vi "Periodic Tasks.vi"(8 "error in":errorcluster) -> ()   [LabVIEW 2018]
doc: "This VI runs in parallel to other tasks. It can contain as many user-defined periodic loops as you need. These can carry out PID or other sorts of timed response."
uses:
  State Machines/Intake.ctl
  State Machines/Climber.ctl
  <vilib>/Rock Robotics/WPI/Solenoid/WPI_SolenoidValue.ctl
  <vilib>/Rock Robotics/WPI/ThirdParty/Phoenix-LabVIEW/Motor Controller/Controls/CTRE_Phoenix_MotorControl_ControlMode.ctl
  <vilib>/Rock Robotics/WPI/ThirdParty/Sensors/navX/_TypeDefs/FRIC_navX_DeviceNumbersTypeDef.ctl
  <vilib>/Rock Robotics/WPI/DriverStation/WPI_DriverStationRobotMode2.ctl
  Robot Global Data.vi
  Support Code/Valkyrie1Buttons.vi
  <vilib>/Rock Robotics/WPI/Utilities/WPI_GetSetVariantRefNum.vi
  <vilib>/Rock Robotics/WPI/Solenoid/WPI_SolenoidSetEnum.vi
  <vilib>/Rock Robotics/Network Tables/NT Write Number.vi
  <vilib>/Rock Robotics/Network Tables/NT Write Boolean.vi
panel:
  in  "ScoreHatchHeight":dbl=1.0
  in  "HP_Height":dbl=1.5
  in  "HatchGetSpeed":dbl=-1.0
  in  "SetpointElevatorCargo":dbl=5.5
  in  "ElevatorCargoDelay":dbl
  in  "Delay Cargo IR":dbl=5.0
  in  "Time to wait":dbl
  in  "Back Timer":dbl=15.0 format="%#_13g"
  in  "Retract back Speed 2":dbl=-0.4 format="%#_13g"
  in  "Retract Speed 2":dbl=-0.3
  in  "Retract Distance 2":dbl=700.0 format="%#_13g"
  in  "Back Speed 2":dbl=0.8
  in  "Front Speed 2":dbl=1.0
  in  "Front Limit 2":dbl=700.0 format="%#_13g"
  in  "Break speed 2":dbl=0.2 format="%#_13g"
  out "Climber State 2":T1=enum."Wait for Start"
  in  "Climb Height":dbl=2.0
  in  "Score Hatch Angle 2":dbl=2.0
  out "Climber State":T1=enum."Wait for Start"
  in  "Retract back Speed":dbl=-0.4 format="%#_13g"
  in  "Retract Distance":dbl=1750.0 format="%#_13g"
  in  "Retract Speed":dbl=-0.3
  in  "Break speed":dbl=0.2 format="%#_13g"
  in  "Front Limit":dbl=1750.0 format="%#_13g"
  in  "Front Speed":dbl=1.0
  in  "Back Speed":dbl=0.75
  out "Encoder Climber":i32
  in  "Score Angle 2nd":dbl=3.0
  in  "Slow Mode":dbl=0.4
  in  "Cargo Deploy angle 2nd Floor":dbl=5.0
  in  "Cargo 2nd Floor Rocket":dbl=9.5
  in  "Cargo ship height":dbl=9.0
  in  "Cargo 1st Floor Rocket":dbl=5.0 format="%#_13g"
  out "elavador  pos":dbl
  in  "Height  Hatch 2nd":dbl=9.0
  out "Intake pos":dbl=23.023681640625
  in  "Turn on point multiplier":dbl=0.6 format="%#_13g"
  in  "Sensitivty":dbl=1.1 format="%#_13g"
  in  "Height Cargo Station":dbl=2.0
  in  "Height Cargo HP":dbl=9.0
  in  "Floor Angle Cargo":dbl=22.0
  in  "Gains":T2={"proportional gain (Kc)"=0.5, "integral time (Ti, min)"=0.1, "derivative time (Td, min)"=0.0} {"derivative time (Td, min)" format="%.3f"; "integral time (Ti, min)" format="%.3f"; "proportional gain (Kc)" format="%.3f"}
  in  "Range":cluster{"output high":dbl, "output low":dbl}={"output high"=1.0, "output low"=-0.4} {"output low" format="%.2f"; "output high" format="%.2f"}
  in  "Disable Range":dbl
  in  "Integral Range":dbl=1.0
  in  "CargoTime":dbl=10.0
  in  "Default height":dbl=3.0 format="%#_13g"
  in  "Cargo Deploy Angle":dbl=15.0
  in  "Tempo de coleta":dbl=7.0 format="%#_13g"
  out "Estado Intake":T3
  in  "Score Hatch Angle":dbl=2.0 format="%#_13g"
  in  "Floor Angle":dbl=23.0
  in  "Hatch intake Speed Floor":dbl=-1.0
  in  "Holding Angle":dbl=4.0
  in  "HP Angle":dbl=1.0 format="%#_13g"
  in  "Intake Arm PID Constants":T4={"P Gain"=0.15, "I Gain"=1e-05, "D Gain"=5.0, "F Gain"=0.0, "I Zone"=10.0, "Min Output"=-0.2999999999999998, "Max Output"=0.3} {"Max Output" min=-1.0 max=1.0 step=0.01; "Min Output" min=-1.0 max=1.0 step=0.01; "I Zone" step=0.01; "F Gain" step=0.01; "D Gain" step=0.01; "I Gain" step=0.01; "P Gain" min=0.0 step=0.01}
  # "Angles"
  # "Intake Control"
  # "Elevator Control"
  # "Climber"
  # "Drivetrain"
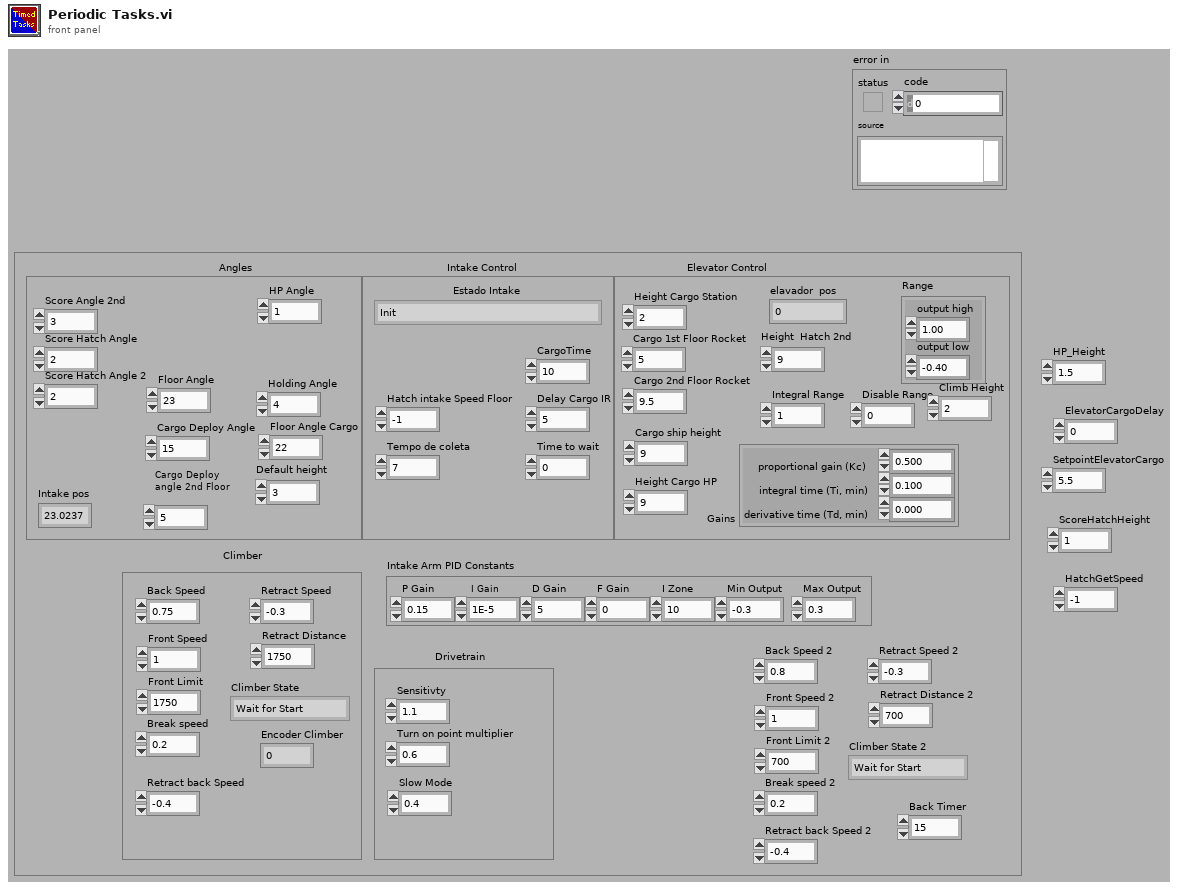
[diagram p1: front panel]
types:
  T1 = typedef "Climber.ctl" = enum16{"Engaging Climb", "Wait for Start", "ELEVATE!", "Hold position", "Forward", "Retract varetas", "Charge", "Sobe so um poquinho", "cabou"}
  T2 = cluster{"proportional gain (Kc)":dbl, "integral time (Ti, min)":dbl, "derivative time (Td, min)":dbl}
  T3 = typedef "Intake.ctl" = enum16{"Init", "Preparar Coletar HP", "Coletar Cargo", "Segurando Cargo", "Preparar Score Cargo", "Score Cargo", "Coletar HP", "Coletar Hatch Chão", "Segurando Hatch", "Preparar Score Hatch", "Score Hatch", "Wait"}
  T4 = cluster{"P Gain":dbl, "I Gain":dbl, "D Gain":dbl, "F Gain":dbl, "I Zone":dbl, "Min Output":dbl, "Max Output":dbl}
  T5 = typedef "WPI_MotorControlDeviceRef.ctl" = cluster{"DeviceStatus":errorcluster, "Type":T6, "PWM":cluster{"PWM Channel":T7, "DeadBand":T8}, "CAN":cluster{"Device Number":u8, "SetOutput VI Ref":variant, "GetOutput VI Ref":variant, "Enable VI Ref":variant, "Disable VI Ref":variant, "Data":variant}, "Invert":bool, "DIO PWM":cluster{"PWM \"Enable\" Channel":T7, "DIOChannel":T9, "PWM Rate":dbl}}
  T6 = typedef "WPI_MotorControlType.ctl" = enum16{"PWM", "CAN", "DIO PWM"}
  T7 = typedef "FPGA_DIOPWMChannel.ctl" = enum8{"PWM 0", "PWM 1", "PWM 2", "PWM 3", "PWM 4", "PWM 5", "PWM 6", "PWM 7", "PWM 8", "PWM 9", "PWM MXP 0", "PWM MXP 1", "PWM MXP 2", "PWM MXP 3", "PWM MXP 4", "PWM MXP 5", "PWM MXP 6", "PWM MXP 7", "PWM MXP 8", "PWM MXP 9", "Invalid"}
  T8 = typedef "WPI_PWMDeadband.ctl" = cluster{"Name":string, "maxPositivePwm":i32, "minPositivePwm":i32, "centerPwm":i32, "maxNegativePwm":i32, "minNegativePwm":i32, "angularRange":u16}
  T9 = typedef "FPGA_DIOChannel.ctl" = enum8{"DIO 0", "DIO 1", "DIO 2", "DIO 3", "DIO 4", "DIO 5", "DIO 6", "DIO 7", "DIO 8", "DIO 9", "DIO MXP 0", "DIO MXP 1", "DIO MXP 2", "DIO MXP 3", "DIO MXP 4", "DIO MXP 5", "DIO MXP 6", "DIO MXP 7", "DIO MXP 8", "DIO MXP 9", "DIO MXP 10", "DIO MXP 11", "DIO MXP 12", "DIO MXP 13", "DIO MXP 14", "DIO MXP 15", "SPI Port CS1", "SPI Port CS2", "SPI Port CS3", "SPI Port MISO", "SPI Port MOSI", "Invalid"}
  T10 = typedef "Button Cluster.ctl" = cluster{"Buttons[0]":bool, "Buttons[1]":bool, "Buttons[2]":bool, "Buttons[3]":bool, "Buttons[4]":bool, "Buttons[5]":bool, "Buttons[6]":bool, "Buttons[7]":bool, "Buttons[8]":bool, "Buttons[9]":bool}
  T11 = typedef "WPI_SwitchDevRef.ctl" = cluster{"DevStatus":errorcluster, "DIO Channel":T9, "CntIndex":T12, "Normally Closed":bool}
  T12 = typedef "FPGA_CounterCtrSystemIndex.ctl" = enum8{"Ctr 0", "Ctr 1", "Ctr 2", "Ctr 3", "Ctr 4", "Ctr 5", "Ctr 6", "Ctr 7", "Invalid"}
  T13 = typedef "WPI_SolenoidDevRef.ctl" = cluster{"DevStatus":errorcluster, "Pneumatics Control Module":u8, "Forward Solenoid Channel":T14, "Reverse Solenoid Channel":T14}
  T14 = typedef "WPI_SolenoidChannel.ctl" = enum8{"Solenoid 0", "Solenoid 1", "Solenoid 2", "Solenoid 3", "Solenoid 4", "Solenoid 5", "Solenoid 6", "Solenoid 7", "Invalid"}
  T15 = typedef "WPI_EncoderDevRef.ctl" = cluster{"DevStatus":errorcluster, "EncoderIndex":T16, "CounterIndex":T12, "DistancePerCount":dbl, "Decoding Type":T17}
  T16 = typedef "FPGA_EncoderIdx.ctl" = enum8{"Enc 0", "Enc 1", "Enc 2", "Enc 3", "Enc 4", "Enc 5", "Enc 6", "Enc 7", "Invalid"}
  T17 = typedef "WPI_EncoderType.ctl" = enum16{"1x", "2x", "4x"}
  T18 = typedef "WPI_SolenoidValue.ctl" = enum16{"Off", "On", "Forward", "Reverse"}
  T19 = typedef "CTRE_Phoenix_MotorControl_ControlMode.ctl" = u16
  T20 = typedef "WPI_CounterDevRef.ctl" = cluster{"DevStatus":errorcluster, "CntIndex":T12}
  T21 = typedef "FRIC_navX_DeviceNumbersTypeDef.ctl" = enum16{"Dev0", "Dev1", "Dev2", "Dev3"}
  T22 = cluster{"Yaw":dbl, "Roll":dbl, "Pitch":dbl, "Heading":dbl, "Fused Heading":dbl}
  T23 = typedef "WPI_RobotDriveDevRef.ctl" = cluster{"DevStatus":errorcluster, "Motors[]":T5[], "Square Inputs":bool, "Max Output":dbl}
  T24 = typedef "Axes Cluster.ctl" = cluster{"Axes[0]":dbl, "Axes[1]":dbl, "Axes[2]":dbl, "Axes[3]":dbl, "Axes[4]":dbl, "Axes[5]":dbl, "Axes[6]":dbl, "Axes[7]":dbl, "Axes[8]":dbl}
  T25 = typedef "WPI_DriverStationRobotMode2.ctl" = enum16{"Autonomous Disabled", "Autonomous Enabled", "Teleop Disabled", "Teleop Enabled", "Disconnected", "Finish", "Test Disabled", "Test Enabled", "Emergency Stopped"}
  T26 = typedef "WPI_CompressorDevRef.ctl" = cluster{"DevStatus":errorcluster, "Pneumatics Control Module":u8}
  T27 = typedef "WPI_JoystickDevRef.ctl" = cluster{"Device":T28}
  T28 = typedef "WPI_JoystickDeviceEnum.ctl" = enum16{"USB 0", "USB 1", "USB 2", "USB 3", "USB 4", "USB 5"}
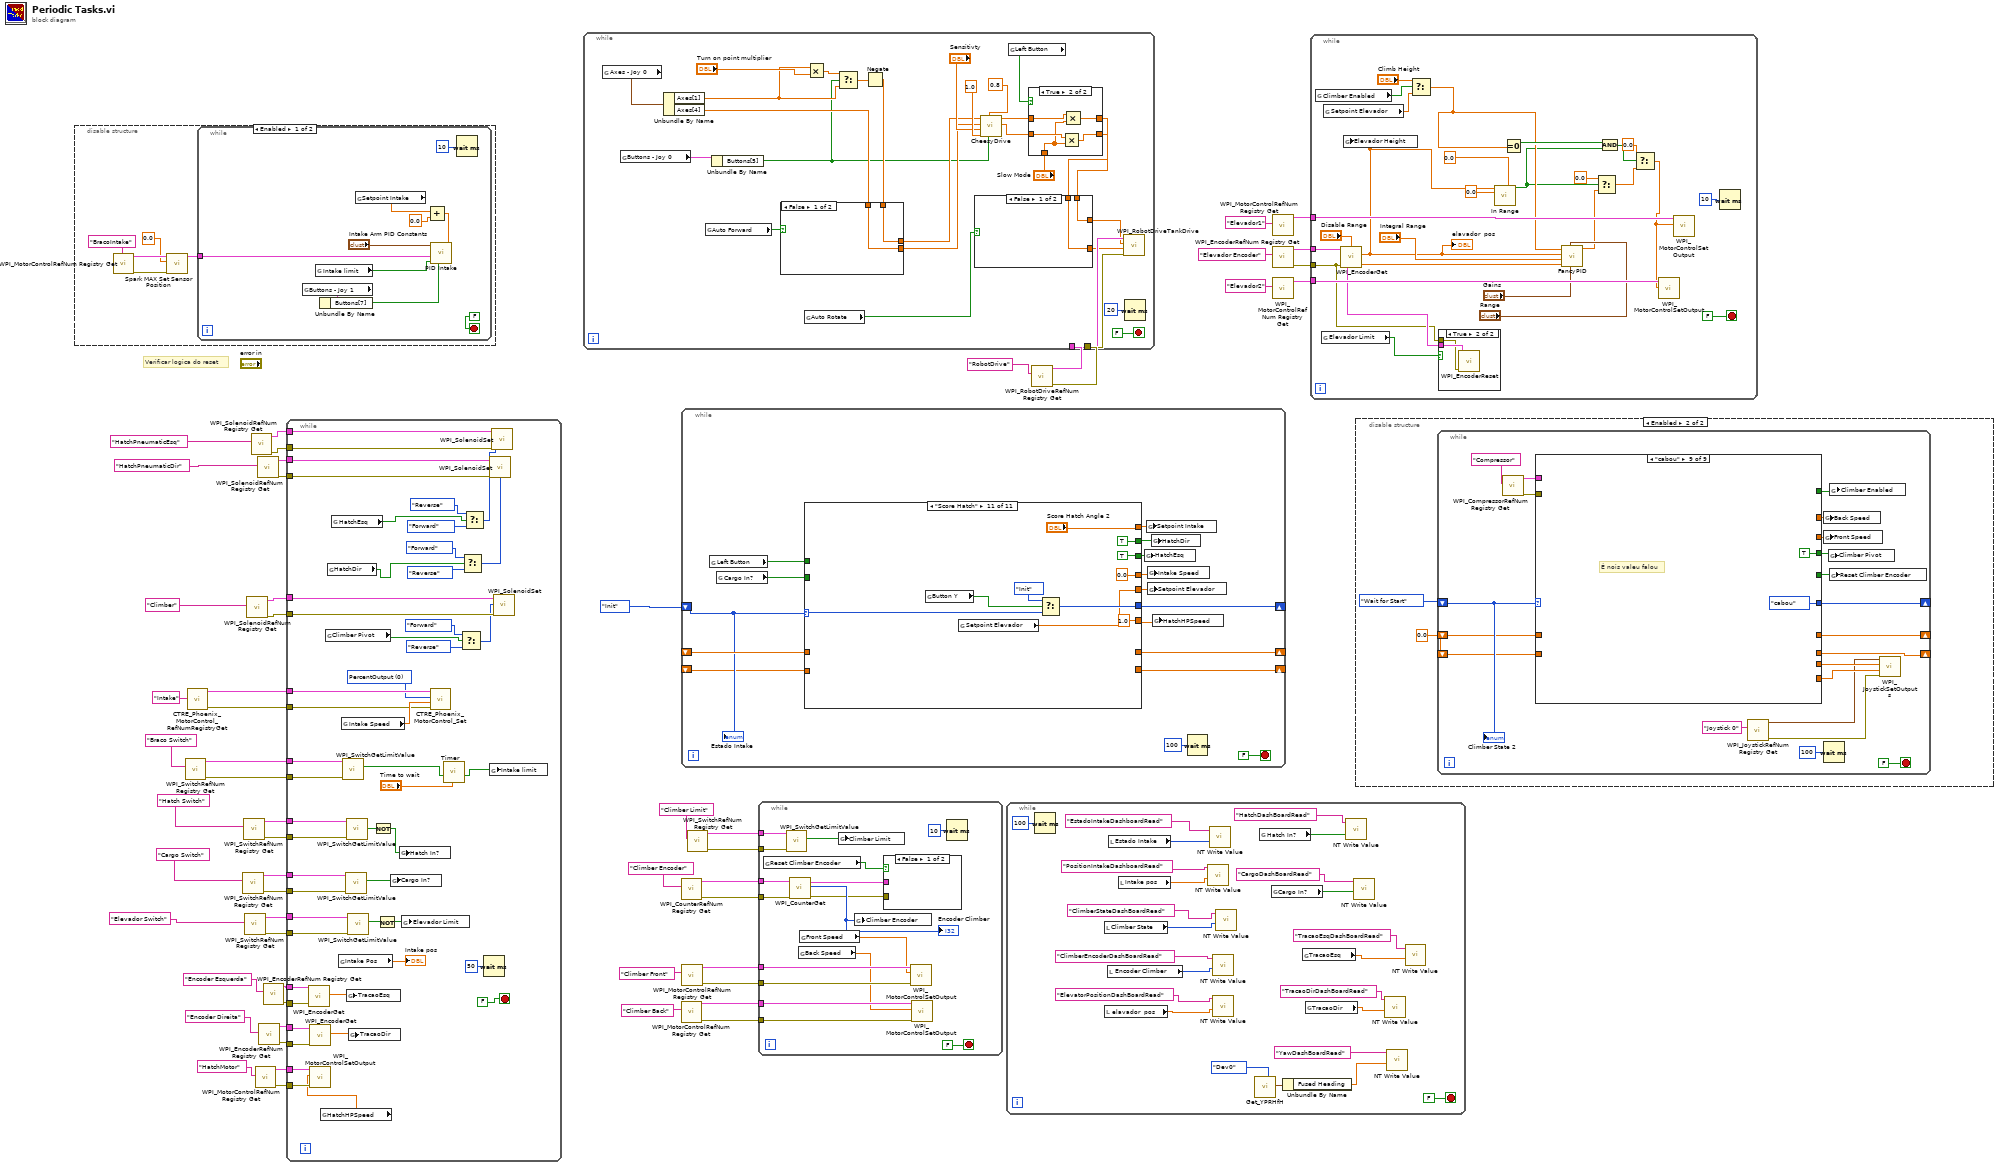
[diagram p0: block diagram]
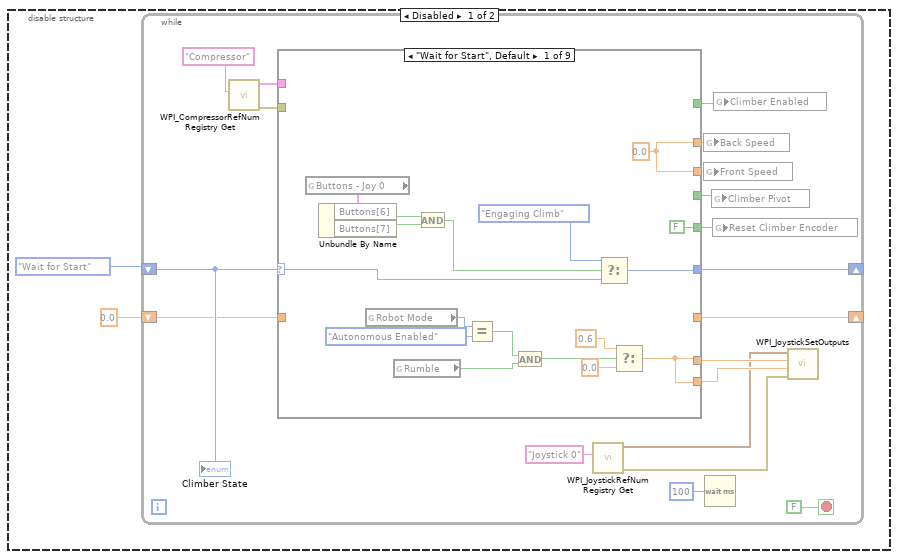
[diagram p2: hidden frame]
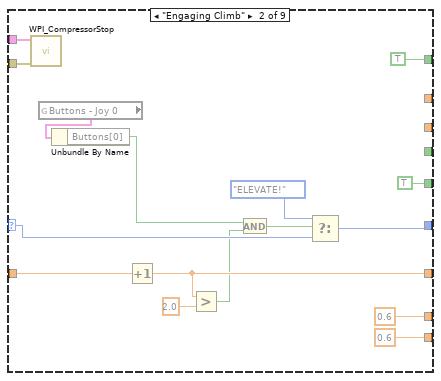
[diagram p3: hidden frame]
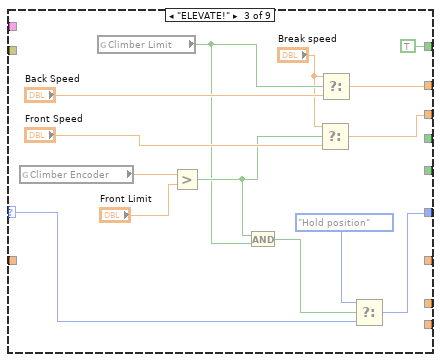
[diagram p4: hidden frame]
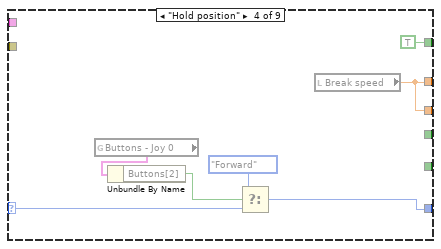
[diagram p5: hidden frame]
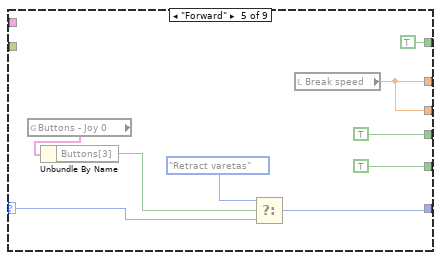
[diagram p6: hidden frame]
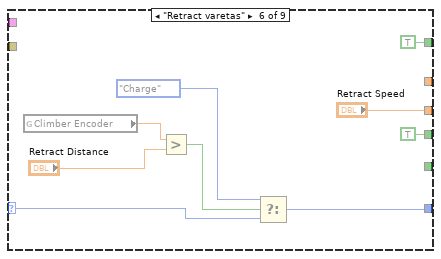
[diagram p7: hidden frame]
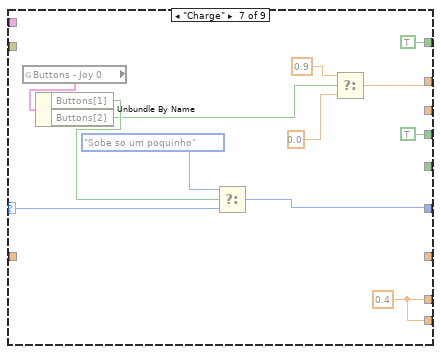
[diagram p8: hidden frame]
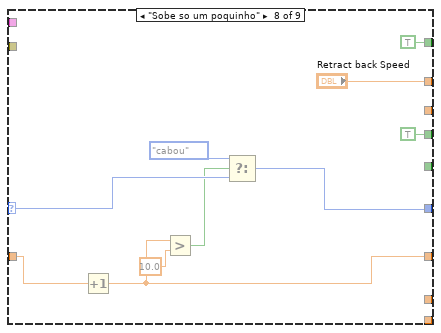
[diagram p9: hidden frame]
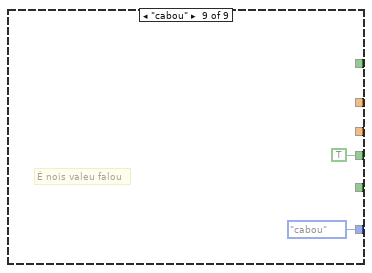
[diagram p10: hidden frame]
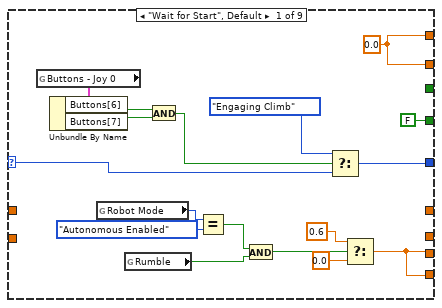
[diagram p11: hidden frame]
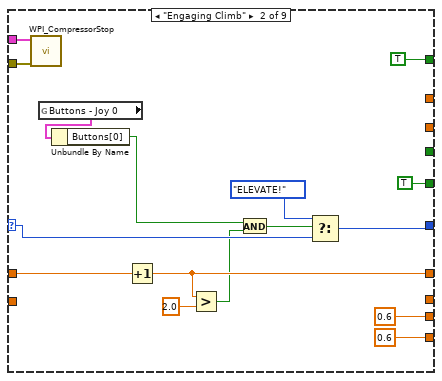
[diagram p12: hidden frame]
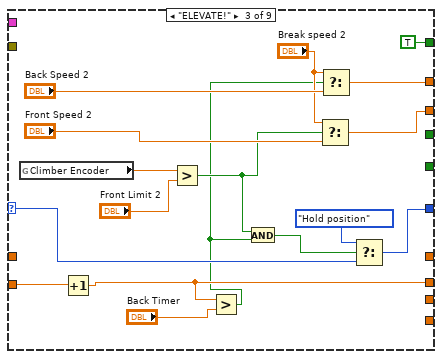
[diagram p13: hidden frame]
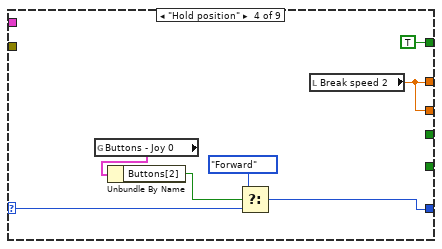
[diagram p14: hidden frame]
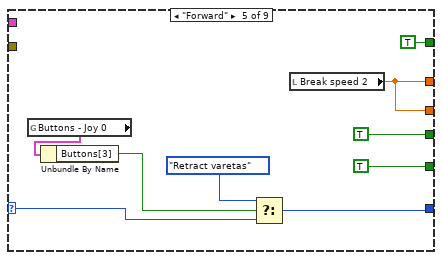
[diagram p15: hidden frame]
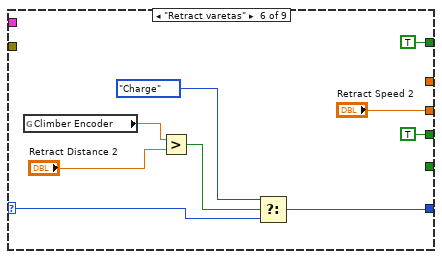
[diagram p16: hidden frame]
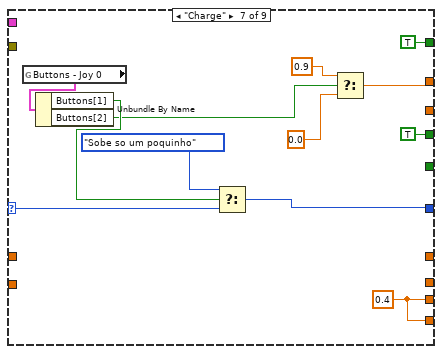
[diagram p17: hidden frame]
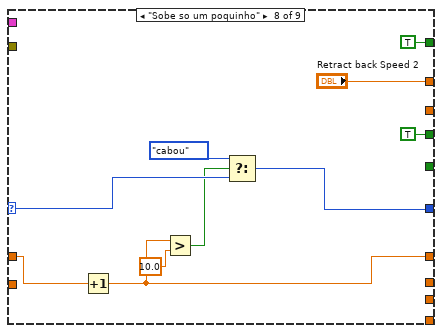
[diagram p18: hidden frame]
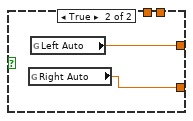
[diagram p20: hidden frame]
diagram:
  # "Verificar logica do reset"
  n1 = disable-structure shown="Enabled" {
    frame Enabled {
      n2 = call <vilib>:"WPI_MotorControlRefNum Registry Get.vi"("refnum name"="BracoIntake") -> ("error out"=w58:errorcluster, "MotorControlDevRef"=w59:T5)  [unwired: 9 in]
      n3 = call <vilib>:"Spark MAX Set Sensor Position.vi"("error in"=w58, "Position"=0.0, "MotorControlDeviceRef"=w59) -> ("MotorControlDeviceRef"=w60:T5)  [unwired: 7 in, 1 out]
      n4 = while {
        tunnel: w60 -> [w69]
        stop <- FALSE stop-if-true
        n5 = global read "Robot Global Data.vi" "Buttons - Joy 1"() -> (w67:T10)
        n6 = global read "Robot Global Data.vi" "Intake limit"() -> (w65:bool)
        n7 = Unbundle By Name(w67) -> ("Buttons[7]"=w66:bool)
        n8 = global read "Robot Global Data.vi" "Setpoint Intake"() -> (w64:dbl)
        n9 = Add(x=w64, y=0.0) -> (x+y=w63:dbl)
        n10 = call "PID Intake.vi"("Encoder Overide"=w66, "Limit"=w65, "Setpoint Intake"=w63, "MotorControlDevRef"=w69, "PID Constants"="Intake Arm PID Constants") -> ()  [unwired: 7 in]
        n11 = Wait (ms)(milliseconds to wait=u32 10) -> ()  [unwired: 1 out]
      }
    }
    frame Disabled {
    }
  }
  n12 = call <vilib>:"WPI_SwitchRefNum Registry Get.vi"("refnum name"="Braco Switch") -> ("error out"=w52:errorcluster, "SwitchDevRef"=w53:T11)  [unwired: 9 in]
  n13 = call <vilib>:"CTRE_Phoenix_MotorControl_RefNumRegistryGet.vi"("refnum name"="Intake") -> ("error out"=w48:errorcluster, "PhoenixMotorControlDevRef"=w49:T5)  [unwired: 9 in]
  n14 = call <vilib>:"WPI_SwitchRefNum Registry Get.vi"("refnum name"="Cargo Switch") -> ("error out"=w39:errorcluster, "SwitchDevRef"=w40:T11)  [unwired: 9 in]
  n15 = call <vilib>:"WPI_SwitchRefNum Registry Get.vi"("refnum name"="Hatch Switch") -> ("error out"=w47:errorcluster, "SwitchDevRef"=w46:T11)  [unwired: 9 in]
  n16 = call <vilib>:"WPI_SwitchRefNum Registry Get.vi"("refnum name"="Elevador Switch") -> ("error out"=w27:errorcluster, "SwitchDevRef"=w26:T11)  [unwired: 9 in]
  n17 = call <vilib>:"WPI_SolenoidRefNum Registry Get.vi"("refnum name"="Climber") -> ("error out"=w43:errorcluster, "SolenoidDevRef"=w42:T13)  [unwired: 9 in]
  n18 = call <vilib>:"WPI_SolenoidRefNum Registry Get.vi"("refnum name"="HatchPneumaticEsq") -> ("error out"=w37:errorcluster, "SolenoidDevRef"=w36:T13)  [unwired: 9 in]
  n19 = call <vilib>:"WPI_MotorControlRefNum Registry Get.vi"("refnum name"="HatchMotor") -> ("error out"=w2:errorcluster, "MotorControlDevRef"=w3:T5)  [unwired: 9 in]
  n20 = call <vilib>:"WPI_SolenoidRefNum Registry Get.vi"("refnum name"="HatchPneumaticDir") -> ("error out"=w54:errorcluster, "SolenoidDevRef"=w55:T13)  [unwired: 9 in]
  n21 = call <vilib>:"WPI_EncoderRefNum Registry Get.vi"("refnum name"="Encoder Direita") -> ("error out"=w4:errorcluster, "EncoderDevRef"=w5:T15)  [unwired: 9 in]
  n22 = call <vilib>:"WPI_EncoderRefNum Registry Get.vi"("refnum name"="Encoder Esquerda") -> ("error out"=w7:errorcluster, "EncoderDevRef"=w8:T15)  [unwired: 9 in]
  n23 = while {
    tunnel: w36 -> [w121]
    tunnel: w37 -> [w120]
    tunnel: w55 -> [w119]
    tunnel: w54 -> [w118]
    tunnel: w42 -> [w117]
    tunnel: w43 -> [w116]
    tunnel: w49 -> [w104]
    tunnel: w53 -> [w101]
    tunnel: w52 -> [w100]
    tunnel: w48 -> [w99]
    tunnel: w46 -> [w97]
    tunnel: w47 -> [w98]
    tunnel: w40 -> [w93]
    tunnel: w39 -> [w92]
    tunnel: w26 -> [w87]
    tunnel: w27 -> [w88]
    tunnel: w7 -> [w84]
    tunnel: w5 -> [w82]
    tunnel: w4 -> [w81]
    tunnel: w8 -> [w79]
    tunnel: w3 -> [w74]
    tunnel: w2 -> [w73]
    stop <- FALSE stop-if-true
    w103 = T19 0 items=["PercentOutput"=0, "Position"=1, "Velocity"=2, "Current"=3, "Follower"=5, "MotionProfile"=6, "MotionMagic"=7, "MotionProfileArc"=10, "Disabled"=15] ("Control Mode")
    n24 = call <vilib>:"WPI_EncoderGet.vi"("error in (no error)"=w84, "EncoderDevRef"=w79) -> ("Distance"=w83:dbl)  [unwired: 4 in, 5 out]
    n25 = call <vilib>:"WPI_EncoderGet.vi"("error in (no error)"=w81, "EncoderDevRef"=w82) -> ("Distance"=w80:dbl)  [unwired: 4 in, 5 out]
    n26 = global read "Robot Global Data.vi" "HatchHPSpeed"() -> (w72:dbl)
    n27 = call <vilib>:"WPI_MotorControlSetOutput.vi"("error in (no error)"=w73, "Output"=w72, "MotorControlDevRef"=w74) -> ()  [unwired: 6 in, 3 out]
    n28 = global read "Robot Global Data.vi" "Climber Pivot"() -> (w105:bool)
    n29 = global read "Robot Global Data.vi" "HatchDir"() -> (w95:bool)
    n30 = global read "Robot Global Data.vi" "HatchEsq"() -> (w94:bool)
    n31 = global read "Robot Global Data.vi" "Intake Pos"() -> (→"Intake pos":dbl)
    n32 = global read "Robot Global Data.vi" "Intake Speed"() -> (w102:dbl)
    n33 = call <vilib>:"WPI_SwitchGetLimitValue.vi"("error in (no error)"=w100, "SwitchDevRef"=w101) -> ("Switch Pressed"=w77:bool)  [unwired: 7 in, 2 out]
    n34 = call <vilib>:"WPI_SwitchGetLimitValue.vi"("error in (no error)"=w92, "SwitchDevRef"=w93) -> ("Switch Pressed"=w85:bool)  [unwired: 7 in, 2 out]
    n35 = call <vilib>:"WPI_SwitchGetLimitValue.vi"("error in (no error)"=w98, "SwitchDevRef"=w97) -> ("Switch Pressed"=w96:bool)  [unwired: 7 in, 2 out]
    n36 = global write "Robot Global Data.vi" "TracaoEsq"(w83) -> ()
    n37 = call <vilib>:"WPI_SwitchGetLimitValue.vi"("error in (no error)"=w88, "SwitchDevRef"=w87) -> ("Switch Pressed"=w89:bool)  [unwired: 7 in, 2 out]
    n38 = global write "Robot Global Data.vi" "TracaoDir"(w80) -> ()
    n39 = Not(x=w96) -> (.not. x?=w91:bool)
    n40 = Not(x=w89) -> (.not. x?=w86:bool)
    n41 = global write "Robot Global Data.vi" "Cargo In?"(w85) -> ()
    n42 = global write "Robot Global Data.vi" "Hatch In?"(w91) -> ()
    n43 = global write "Robot Global Data.vi" "Elevador Limit"(w86) -> ()
    n44 = call <vilib>:"CTRE_Phoenix_MotorControl_Set.vi"("error in (no error)"=w99, "Output"=w102, "Control Mode"=w103, "PhoenixMotorControlDevRef"=w104) -> ()  [unwired: 6 in, 2 out]
    n45 = call "Timer.vi"("Timer to wait"="Time to wait", "Switch Pressed"=w77) -> ("Out"=w76:bool)  [unwired: 9 in]
    n46 = Select(t=WPI_SolenoidValue."Forward" ("Value"), s=w105, f=WPI_SolenoidValue."Reverse") -> (s? t:f=w111:T18)
    n47 = Select(t=WPI_SolenoidValue."Forward" ("Value"), s=w95, f=WPI_SolenoidValue."Reverse") -> (s? t:f=w108:T18)
    n48 = Select(t=WPI_SolenoidValue."Reverse" ("Value"), s=w94, f=WPI_SolenoidValue."Forward") -> (s? t:f=w75:T18)
    n49 = Wait (ms)(milliseconds to wait=u32 50) -> ()  [unwired: 1 out]
    n50 = call-poly <vilib>:"WPI_SolenoidSet.vi"("error in (no error)"=w118, "Value"=w108, "SolenoidDevRef"=w119) -> ()  [unwired: 7 in, 2 out]
    n51 = global write "Robot Global Data.vi" "Intake limit"(w76) -> ()
    n52 = call-poly <vilib>:"WPI_SolenoidSet.vi"("error in (no error)"=w120, "Value"=w75, "SolenoidDevRef"=w121) -> ()  [unwired: 7 in, 2 out]
    n53 = call-poly <vilib>:"WPI_SolenoidSet.vi"("error in (no error)"=w116, "Value"=w111, "SolenoidDevRef"=w117) -> ()  [unwired: 7 in, 2 out]
  }
  n54 = call <vilib>:"WPI_CounterRefNum Registry Get.vi"("refnum name"="Climber Encoder") -> ("error out"=w19:errorcluster, "CounterDevRef"=w20:T20)  [unwired: 9 in]
  n55 = call <vilib>:"WPI_MotorControlRefNum Registry Get.vi"("refnum name"="Climber Back") -> ("error out"=w13:errorcluster, "MotorControlDevRef"=w15:T5)  [unwired: 9 in]
  n56 = while {
    shift-right: [w136] -> _
    shift-left: Intake."Init" -> [w132]
    shift-right: [w133] -> _
    shift-left: _ -> [w134]
    shift-right: [w131] -> _
    shift-left: _ -> [w130]
    stop <- FALSE stop-if-true
    n57 = global read "Valkyrie1Buttons.vi" "Left Button"() -> (w123:bool)
    n58 = global read "Robot Global Data.vi" "Cargo In?"() -> (w124:bool)
    n59 = case shown="\"Score Hatch\"" w132 {
      selector: w132 -> [w162 w178 w202 w219 w233 w256 w263 w272 w286 w310 w319]
      tunnel: [w142 "Floor Angle Cargo" w195 w207 w239 "HP Angle" _ "Floor Angle" "Holding Angle" w299 "Score Hatch Angle 2"] -> w129
      tunnel: [FALSE FALSE FALSE FALSE FALSE TRUE FALSE FALSE TRUE TRUE TRUE] -> w128
      tunnel: [FALSE FALSE FALSE FALSE FALSE TRUE FALSE FALSE TRUE TRUE TRUE] -> w127
      tunnel: [w151 w179 w192 w205 w235 w254 w266 w275 w290 w307 w318] -> w136
      tunnel: w134 -> [_ _ _ _ w230 w246 _ _ _ _ _]
      tunnel: [_ _ _ _ w228 w251 _ _ _ _ _] -> w133
      tunnel: [0.0 ("Hatch intake Speed Floor") 1.0 ("Hatch intake Speed Floor") w201 0.0 ("Hatch intake Speed Floor") -1.0 ("Hatch intake Speed Floor") 0.0 ("Hatch intake Speed Floor") _ "Hatch intake Speed Floor" 0.0 ("Hatch intake Speed Floor") 0.0 ("Hatch intake Speed Floor") 0.0 ("Hatch intake Speed Floor")] -> w126
      tunnel: w123 -> [w143 _ w188 _ _ _ _ w269 w283 _ _]
      tunnel: [_ _ _ _ _ 0.0 ("y") w259 _ _ _ _] -> w131
      tunnel: w130 -> [_ _ _ _ _ _ w260 _ _ _ _]
      tunnel: [0.0 ("ElevadorRocket") w187 0.0 ("ElevadorRocket") w212 w231 "HP_Height" 0.0 ("ElevadorRocket") 0.0 ("ElevadorRocket") 0.0 ("ElevadorRocket") w302 w313] -> w125
      tunnel: w124 -> [w148 w170 w200 _ _ _ _ _ _ _ _]
      tunnel: [_ _ _ _ _ "HatchGetSpeed" 0.1 ("HatchGetSpeed") 0.1 ("HatchSpeed") w281 -0.1 ("HatchGetSpeed") 1.0 ("HatchGetSpeed")] -> w122
      frame "Init", Default {
        n60 = global read "Valkyrie1Buttons.vi" "Button A"() -> (w152:bool)
        n61 = global read "Valkyrie1Buttons.vi" "Button X"() -> (w154:bool)
        n62 = global read "Valkyrie1Buttons.vi" "Button B"() -> (w153:bool)
        n63 = call "Timer.vi"("Timer to wait"="Delay Cargo IR", "Switch Pressed"=w143) -> ("Out"=w144:bool)  [unwired: 9 in]
        n64 = global read "Robot Global Data.vi" "Elevador Height"() -> (w139:dbl)
        n65 = Select(t=Intake."Preparar Coletar HP", s=w152, f=w162) -> (s? t:f=w161:T3)
        n66 = Select(t=Intake."Coletar Hatch Chão", s=w154, f=w161) -> (s? t:f=w156:T3)
        n67 = Less?(x=w139, y=6.0) -> (x < y?=w141:bool)
        n68 = Select(t=Intake."Coletar Cargo", s=w153, f=w156) -> (s? t:f=w150:T3)
        n69 = Select(t="Default height", s=w141, f=4.0) -> (s? t:f=w142:dbl)
        n70 = Select(t=Intake."Segurando Hatch", s=w144, f=w150) -> (s? t:f=w149:T3)
        n71 = Select(t=Intake."Segurando Cargo", s=w148, f=w149) -> (s? t:f=w151:T3)
      }
      frame "Coletar Cargo" {
        n72 = global read "Robot Global Data.vi" "Intake Pos"() -> (w168:dbl)
        n73 = global read "Valkyrie1Buttons.vi" "Down"() -> (w176:bool)
        n74 = global read "Valkyrie1Buttons.vi" "Up"() -> (w177:bool)
        n75 = Greater Or Equal?(x=w168, y=20.0) -> (x >= y?=w166:bool)
        n76 = And(x=w170, y=w166) -> (x .and. y?=w169:bool)
        n77 = global read "Valkyrie1Buttons.vi" "Button Y"() -> (w175:bool)
        n78 = Select(t=Intake."Segurando Cargo", s=w169, f=w178) -> (s? t:f=w180:T3)
        n79 = Select(t="Height Cargo Station", s=w176, f=0.0) -> (s? t:f=w186:dbl)
        n80 = Select(t="Height Cargo HP", s=w177, f=w186) -> (s? t:f=w187:dbl)
        n81 = Select(t=Intake."Init", s=w175, f=w180) -> (s? t:f=w179:T3)
      }
      frame "Segurando Cargo" {
        n82 = global read "Valkyrie1Buttons.vi" "Button Y"() -> (w190:bool)
        n83 = Select(t=Intake."Preparar Score Cargo", s=w188, f=w202) -> (s? t:f=w191:T3)
        n84 = local read "Holding Angle"() -> (w195:dbl)
        n85 = Select(t=Intake."Init", s=w190, f=w191) -> (s? t:f=w192:T3)
        n86 = Select(t=0.0, s=w200, f=0.1) -> (s? t:f=w201:dbl)
      }
      frame "Preparar Score Cargo" {
        n87 = global read "Valkyrie1Buttons.vi" "Up"() -> (w208:bool)
        n88 = global read "Valkyrie1Buttons.vi" "Down"() -> (w211:bool)
        n89 = global read "Valkyrie1Buttons.vi" "Right Button"() -> (w217:bool)
        n90 = global read "Valkyrie1Buttons.vi" "Button Y"() -> (w204:bool)
        n91 = Select(t=Intake."Score Cargo", s=w217, f=w219) -> (s? t:f=w206:T3)
        n92 = Select(t=Intake."Init", s=w204, f=w206) -> (s? t:f=w205:T3)
        n93 = Select(t="Cargo ship height", s=w211, f="Cargo 1st Floor Rocket") -> (s? t:f=w215:dbl)
        n94 = Select(t="Cargo Deploy angle 2nd Floor", s=w208, f="Cargo Deploy Angle") -> (s? t:f=w207:dbl)
        n95 = Select(t="Cargo 2nd Floor Rocket", s=w208, f=w215) -> (s? t:f=w212:dbl)
      }
      frame "Score Cargo" {
        n96 = Increment(x=w230) -> (x+1=w228:dbl)
        n97 = Greater?(x=w228, y="CargoTime") -> (0:w225:bool)
        n98 = Greater?(x=w228, y="ElevatorCargoDelay") -> (0:w224:bool)
        n99 = And(x=w225, y=w224) -> (x .and. y?=w223:bool)
        n100 = Select(t=Intake."Init", s=w223, f=w233) -> (s? t:f=w235:T3)
        n101 = global read "Robot Global Data.vi" "Setpoint Elevador"() -> (w227:dbl)
        n102 = local read "Cargo Deploy Angle"() -> (w239:dbl)
        n103 = Select(t=w227, s=w224, f="SetpointElevatorCargo") -> (s? t:f=w231:dbl)
      }
      frame "Preparar Coletar HP" {
        n104 = global read "Valkyrie1Buttons.vi" "Button X"() -> (w241:bool)
        n105 = Increment(x=w246) -> (x+1=w251:dbl)
        n106 = global read "Valkyrie1Buttons.vi" "Button Y"() -> (w243:bool)
        n107 = Greater?(x=w251, y=7.0) -> ()  [unwired: 1 out]
        n108 = Select(t=Intake."Segurando Hatch", s=w241, f=w256) -> (s? t:f=w255:T3)
        n109 = Select(t=Intake."Init", s=w243, f=w255) -> (s? t:f=w254:T3)
      }
      frame "Coletar HP" {
        n110 = Increment(x=w260) -> (x+1=w259:dbl)
        n111 = Greater?(x=w259, y="Tempo de coleta") -> (0:w264:bool)
        n112 = Select(t=Intake."Segurando Hatch", s=w264, f=w263) -> (s? t:f=w266:T3)
      }
      frame "Coletar Hatch Chão" {
        n113 = global read "Valkyrie1Buttons.vi" "Button Y"() -> (w270:bool)
        n114 = Select(t=Intake."Segurando Hatch", s=w269, f=w272) -> (s? t:f=w274:T3)
        n115 = Select(t=Intake."Init", s=w270, f=w274) -> (s? t:f=w275:T3)
      }
      frame "Segurando Hatch" {
        n116 = global read "Valkyrie1Buttons.vi" "Button Y"() -> (w284:bool)
        n117 = Select(t=Intake."Preparar Score Hatch", s=w283, f=w286) -> (s? t:f=w288:T3)
        n118 = Select(t=Intake."Init", s=w284, f=w288) -> (s? t:f=w290:T3)
        n119 = Negate(x=0.2 ("HatchSpeed")) -> (-x=w281:dbl)
      }
      frame "Preparar Score Hatch" {
        n120 = global read "Valkyrie1Buttons.vi" "Up"() -> (w298:bool)
        n121 = global read "Valkyrie1Buttons.vi" "Right Button"() -> (w304:bool)
        n122 = global read "Valkyrie1Buttons.vi" "Button Y"() -> (w303:bool)
        n123 = Select(t=Intake."Score Hatch", s=w304, f=w310) -> (s? t:f=w308:T3)
        n124 = Select(t=Intake."Init", s=w303, f=w308) -> (s? t:f=w307:T3)
        n125 = Select(t="Height  Hatch 2nd", s=w298, f="ScoreHatchHeight") -> (s? t:f=w302:dbl)
        n126 = Select(t="Score Angle 2nd", s=w298, f="Score Hatch Angle") -> (s? t:f=w299:dbl)
      }
      frame "Score Hatch" {
        n127 = global read "Valkyrie1Buttons.vi" "Button Y"() -> (w316:bool)
        n128 = global read "Robot Global Data.vi" "Setpoint Elevador"() -> (w313:dbl)
        n129 = Select(t=Intake."Init", s=w316, f=w319) -> (s? t:f=w318:T3)
      }
    }
    n130 = global write "Robot Global Data.vi" "HatchEsq"(w127) -> ()
    n131 = global write "Robot Global Data.vi" "Setpoint Intake"(w129) -> ()
    n132 = global write "Robot Global Data.vi" "Intake Speed"(w126) -> ()
    n133 = global write "Robot Global Data.vi" "Setpoint Elevador"(w125) -> ()
    n134 = global write "Robot Global Data.vi" "HatchDir"(w128) -> ()
    n135 = global write "Robot Global Data.vi" "HatchHPSpeed"(w122) -> ()
    n136 = Wait (ms)(milliseconds to wait=u32 100) -> ()  [unwired: 1 out]
    "Estado Intake" <- w132
  }
  n137 = call <vilib>:"WPI_MotorControlRefNum Registry Get.vi"("refnum name"="Climber Front") -> ("error out"=w14:errorcluster, "MotorControlDevRef"=w16:T5)  [unwired: 9 in]
  n138 = call <vilib>:"WPI_SwitchRefNum Registry Get.vi"("refnum name"="Climber Limit") -> ("error out"=w23:errorcluster, "SwitchDevRef"=w24:T11)  [unwired: 9 in]
  n139 = while {
    tunnel: w24 -> [w337]
    tunnel: w23 -> [w336]
    tunnel: w20 -> [w335]
    tunnel: w19 -> [w334]
    tunnel: w16 -> [w332]
    tunnel: w15 -> [w331]
    tunnel: w14 -> [w330]
    tunnel: w13 -> [w329]
    stop <- FALSE stop-if-true
    n140 = global read "Robot Global Data.vi" "Reset Climber Encoder"() -> (w324:bool)
    n141 = call <vilib>:"WPI_SwitchGetLimitValue.vi"("error in (no error)"=w336, "SwitchDevRef"=w337) -> ("Switch Pressed"=w325:bool)  [unwired: 7 in, 2 out]
    n142 = call <vilib>:"WPI_CounterGet.vi"("error in (no error)"=w334, "CounterDevRef in"=w335) -> ("error out"=w326:errorcluster, "Value"=w333:i32, "CounterDevRef out"=w327:T20)  [unwired: 4 in, 3 out]
    "Encoder Climber" <- w333
    n143 = global read "Robot Global Data.vi" "Back Speed"() -> (w328:dbl)
    n144 = global read "Robot Global Data.vi" "Front Speed"() -> (w323:dbl)
    n145 = global write "Robot Global Data.vi" "Climber Limit"(w325) -> ()
    n146 = global write "Robot Global Data.vi" "Climber Encoder"(w333) -> ()
    n147 = case shown="False" w324 {
      tunnel: w327 -> [_ w341]
      tunnel: w326 -> [_ w340]
      frame False {
      }
      frame True {
        n148 = call <vilib>:"WPI_CounterReset.vi"("error in (no error)"=w340, "CounterDevRef in"=w341) -> ()  [unwired: 8 in, 2 out]
      }
    }
    n149 = call <vilib>:"WPI_MotorControlSetOutput.vi"("error in (no error)"=w330, "Output"=w323, "MotorControlDevRef"=w332) -> ()  [unwired: 6 in, 3 out]
    n150 = call <vilib>:"WPI_MotorControlSetOutput.vi"("error in (no error)"=w329, "Output"=w328, "MotorControlDevRef"=w331) -> ()  [unwired: 6 in, 3 out]
    n151 = Wait (ms)(milliseconds to wait=u32 10) -> ()  [unwired: 1 out]
  }
  n152 = while {
    stop <- FALSE stop-if-true
    n153 = Wait (ms)(milliseconds to wait=u32 100) -> ()  [unwired: 1 out]
    n154 = local read "Climber State"() -> (w352:T1)
    n155 = local read "elavador  pos"() -> (w360:dbl)
    n156 = local read "Encoder Climber"() -> (w358:i32)
    n157 = local read "Estado Intake"() -> (w356:T3)
    n158 = local read "Intake pos"() -> (w354:dbl)
    n159 = call-poly <vilib>:"NT Write Value.vi"("Numeric"=w354, "Name"="PositionIntakeDashboardRead") -> ()  [unwired: 9 in, 1 out]
    n160 = call-poly <vilib>:"NT Write Value.vi"("Numeric"=w356, "Name"="EstadoIntakeDashboardRead") -> ()  [unwired: 9 in, 1 out]
    n161 = call-poly <vilib>:"NT Write Value.vi"("Numeric"=w358, "Name"="ClimberEncoderDashBoardRead") -> ()  [unwired: 9 in, 1 out]
    n162 = call-poly <vilib>:"NT Write Value.vi"("Numeric"=w360, "Name"="ElevatorPositionDashBoardRead") -> ()  [unwired: 9 in, 1 out]
    n163 = call-poly <vilib>:"NT Write Value.vi"("Numeric"=w352, "Name"="ClimberStateDashBoardRead") -> ()  [unwired: 9 in, 1 out]
    n164 = call <vilib>:"Get_YPRHfH.vi"("Device Number"=FRIC_navX_DeviceNumbersTypeDef."Dev0") -> ("YRPHfH"=w345:T22)  [unwired: 10 in]
    n165 = global read "Robot Global Data.vi" "Hatch In?"() -> (w362:bool)
    n166 = global read "Robot Global Data.vi" "Cargo In?"() -> (w365:bool)
    n167 = Unbundle By Name(w345) -> ("Fused Heading"=w344:dbl)
    n168 = global read "Robot Global Data.vi" "TracaoEsq"() -> (w351:dbl)
    n169 = global read "Robot Global Data.vi" "TracaoDir"() -> (w349:dbl)
    n170 = call-poly <vilib>:"NT Write Value.vi"("Boolean"=w362, "Name"="HatchDashBoardRead") -> ()  [unwired: 9 in, 1 out]
    n171 = call-poly <vilib>:"NT Write Value.vi"("Boolean"=w365, "Name"="CargoDashBoardRead") -> ()  [unwired: 9 in, 1 out]
    n172 = call-poly <vilib>:"NT Write Value.vi"("Numeric"=w349, "Name"="TracaoDirDashBoardRead") -> ()  [unwired: 9 in, 1 out]
    n173 = call-poly <vilib>:"NT Write Value.vi"("Numeric"=w344, "Name"="YawDashBoardRead") -> ()  [unwired: 9 in, 1 out]
    n174 = call-poly <vilib>:"NT Write Value.vi"("Numeric"=w351, "Name"="TracaoEsqDashBoardRead") -> ()  [unwired: 9 in, 1 out]
  }
  n175 = call <vilib>:"WPI_RobotDriveRefNum Registry Get.vi"("refnum name"="RobotDrive") -> ("error out"=w12:errorcluster, "RobotDriveDevRef"=w11:T23)  [unwired: 9 in]
  n176 = while {
    tunnel: w12 -> [w390]
    tunnel: w11 -> [w389]
    stop <- FALSE stop-if-true
    n177 = global read "Robot Global Data.vi" "Axes - Joy 0"() -> (w392:T24)
    n178 = global read "Robot Global Data.vi" "Buttons - Joy 0"() -> (w367:T10)
    n179 = Unbundle By Name(w392) -> ("Axes[1]"=w382:dbl, "Axes[4]"=w374:dbl)
    n180 = global read "Robot Global Data.vi" "Auto Forward"() -> (w373:bool)
    n181 = Unbundle By Name(w367) -> ("Buttons[5]"=w366:bool)
    n182 = global read "Robot Global Data.vi" "Auto Rotate"() -> (w368:bool)
    n183 = Multiply(x=w382, y="Turn on point multiplier") -> (x*y=w385:dbl)
    n184 = Select(t=w385, s=w366, f=w382) -> (s? t:f=w383:dbl)
    n185 = Negate(x=w383) -> (-x=w376:dbl)
    n186 = case shown="False" w373 {
      tunnel: [w399 w401] -> w377
      tunnel: [w398 w400] -> w375
      tunnel: w376 -> [w399 _]
      tunnel: w374 -> [w398 _]
      frame False {
      }
      frame True {
        n187 = global read "Robot Global Data.vi" "Throttle Auto"() -> (w401:dbl)
        n188 = global read "Robot Global Data.vi" "Wheel Auto"() -> (w400:dbl)
      }
    }
    n189 = call "CheesyDrive.vi"("Quickturn"=w366, "WheelNonLinearity"=0.8, "negInertiaScalar"=1.0, "Sensitivty"="Sensitivty", "Wheel"=w375, "Throttle"=w377) -> ("Right PWM"=w379:dbl, "Left PWM"=w380:dbl)  [unwired: 4 in]
    n190 = global read "Valkyrie1Buttons.vi" "Left Button"() -> (w381:bool)
    n191 = case shown="True" w381 {
      tunnel: w380 -> [w403 w406]
      tunnel: [w403 w408] -> w370
      tunnel: w379 -> [w402 w405]
      tunnel: [w402 w407] -> w369
      tunnel: "Slow Mode" -> [_ w404]
      frame False {
      }
      frame True {
        n192 = Multiply(x=w405, y=w404) -> (x*y=w407:dbl)
        n193 = Multiply(x=w406, y=w404) -> (x*y=w408:dbl)
      }
    }
    n194 = case shown="False" w368 {
      tunnel: [w395 w397] -> w372
      tunnel: [w394 w396] -> w371
      tunnel: w370 -> [w395 _]
      tunnel: w369 -> [w394 _]
      frame False {
      }
      frame True {
        n195 = global read "Robot Global Data.vi" "Right Auto"() -> (w396:dbl)
        n196 = global read "Robot Global Data.vi" "Left Auto"() -> (w397:dbl)
      }
    }
    n197 = call <vilib>:"WPI_RobotDriveTankDrive.vi"("error in (no error)"=w390, "Right axis value"=w371, "Left axis value"=w372, "RobotDriveDevRef"=w389) -> ()  [unwired: 5 in, 3 out]
    n198 = Wait (ms)(milliseconds to wait=u32 20) -> ()  [unwired: 1 out]
  }
  n199 = call <vilib>:"WPI_MotorControlRefNum Registry Get.vi"("refnum name"="Elevador1") -> ("MotorControlDevRef"=w29:T5)  [unwired: 9 in, 1 out]
  n200 = call <vilib>:"WPI_EncoderRefNum Registry Get.vi"("refnum name"="Elevador Encoder") -> ("error out"=w32:errorcluster, "EncoderDevRef"=w33:T15)  [unwired: 9 in]
  n201 = call <vilib>:"WPI_MotorControlRefNum Registry Get.vi"("refnum name"="Elevador2") -> ("MotorControlDevRef"=w28:T5)  [unwired: 9 in, 1 out]
  n202 = while {
    tunnel: w33 -> [w419]
    tunnel: w32 -> [w418]
    tunnel: w29 -> [w433]
    tunnel: w28 -> [w432]
    stop <- FALSE stop-if-true
    n203 = global read "Robot Global Data.vi" "Climber Enabled"() -> (w413:bool)
    n204 = global read "Robot Global Data.vi" "Elevador Limit"() -> (w420:bool)
    n205 = global read "Robot Global Data.vi" "Setpoint Elevador"() -> (w416:dbl)
    n206 = call <vilib>:"WPI_EncoderGet.vi"("error in (no error)"=w418, "EncoderDevRef"=w419) -> ("Distance"=w417:dbl)  [unwired: 4 in, 5 out]
    "elavador  pos" <- w417
    n207 = global write "Robot Global Data.vi" "Elevador Height"(w417) -> ()
    n208 = Select(t="Climb Height", s=w413, f=w416) -> (s? t:f=w415:dbl)
    n209 = case shown="True" w420 {
      tunnel: w419 -> [_ w436]
      tunnel: w418 -> [_ w435]
      frame False {
      }
      frame True {
        n210 = call <vilib>:"WPI_EncoderReset.vi"("error in (no error)"=w435, "EncoderDevRef"=w436) -> ()  [unwired: 8 in, 2 out]
      }
    }
    n211 = call "In Range.vi"("Range"=0.0, "Setpoint"=0.0, "Value"=w417) -> ("in range?"=w412:bool)  [unwired: 8 in]
    n212 = Equal To 0?(x=w415) -> (x = 0?=w426:bool)
    n213 = call "FancyPID.vi"("Gains"="Gains", "Range"="Range", "Disable Range"="Disable Range", "Integral Range"="Integral Range", "Process variable"=w417, "Setpoint"=w415) -> ("output"=w411:dbl)  [unwired: 5 in]
    n214 = Select(t=0.0, s=w412, f=w411) -> (s? t:f=w410:dbl)
    n215 = And(x=w426, y=w412) -> (x .and. y?=w423:bool)
    n216 = Select(t=0.0, s=w423, f=w410) -> (s? t:f=w421:dbl)
    n217 = call <vilib>:"WPI_MotorControlSetOutput.vi"("Output"=w421, "MotorControlDevRef"=w432) -> ()  [unwired: 7 in, 3 out]
    n218 = call <vilib>:"WPI_MotorControlSetOutput.vi"("Output"=w421, "MotorControlDevRef"=w433) -> ()  [unwired: 7 in, 3 out]
    n219 = Wait (ms)(milliseconds to wait=u32 10) -> ()  [unwired: 1 out]
  }
  n220 = disable-structure shown="Enabled" {
    frame Disabled {
      n221 = while {
        shift-right: [w454] -> _
        shift-left: Climber."Wait for Start" -> [w456]
        shift-right: [w450] -> _
        shift-left: 0.0 -> [w451]
        stop <- FALSE stop-if-true
        n222 = call <vilib>:"WPI_CompressorRefNum Registry Get.vi"("refnum name"="Compressor") -> ("error out"=w441:errorcluster, "CompressorDevRef"=w442:T26)  [unwired: 9 in]
        n223 = case shown="\"Wait for Start\", Default" w456 {
          selector: w456 -> [w470 w484 w497 w509 w517 w525 w539 w549 _]
          tunnel: [w471 w485 w498 w510 w518 w526 w540 w550 Climber."cabou"] -> w454
          tunnel: [w467 _ w504 w511 w519 _ w534 "Retract back Speed" _] -> w453
          tunnel: [w467 _ w502 w511 w519 "Retract Speed" _ _ _] -> w452
          tunnel: w451 -> [_ w490 _ _ _ _ _ w547 _]
          tunnel: [_ w489 _ _ _ _ _ w546 _] -> w450
          tunnel: [w461 0.6 _ _ _ _ w541 _ _] -> w449
          tunnel: [w461 0.6 _ _ _ _ w541 _ _] -> w448
          tunnel: [_ _ _ _ TRUE TRUE TRUE TRUE TRUE] -> w444
          tunnel: [FALSE TRUE _ _ TRUE _ _ _ _] -> w443
          tunnel: w442 -> [_ w477 _ _ _ _ _ _ _]
          tunnel: w441 -> [_ w476 _ _ _ _ _ _ _]
          tunnel: [_ TRUE TRUE TRUE TRUE TRUE TRUE TRUE _] -> w439
          frame "Wait for Start", Default {
            w467 = 0.0
            n224 = global read "Robot Global Data.vi" "Buttons - Joy 0"() -> (w474:T10)
            n225 = Unbundle By Name(w474) -> ("Buttons[6]"=w473:bool, "Buttons[7]"=w472:bool)
            n226 = global read "Robot Global Data.vi" "Robot Mode"() -> (w465:T25)
            n227 = global read "Robot Global Data.vi" "Rumble"() -> (w462:bool)
            n228 = And(x=w473, y=w472) -> (x .and. y?=w468:bool)
            n229 = Equal?(x=w465, y=WPI_DriverStationRobotMode2."Autonomous Enabled") -> (x = y?=w463:bool)
            n230 = And(x=w463, y=w462) -> (x .and. y?=w460:bool)
            n231 = Select(t=Climber."Engaging Climb", s=w468, f=w470) -> (s? t:f=w471:T1)
            n232 = Select(t=0.6, s=w460, f=0.0) -> (s? t:f=w461:dbl)
          }
          frame "Engaging Climb" {
            n233 = call <vilib>:"WPI_CompressorStop.vi"("error in (no error)"=w476, "CompressorDevRef"=w477) -> ()  [unwired: 8 in, 2 out]
            n234 = global read "Robot Global Data.vi" "Buttons - Joy 0"() -> (w482:T10)
            n235 = Unbundle By Name(w482) -> ("Buttons[0]"=w479:bool)
            n236 = Increment(x=w490) -> (x+1=w489:dbl)
            n237 = Greater?(x=w489, y=2.0) -> (0:w480:bool)
            n238 = And(x=w479, y=w480) -> (x .and. y?=w481:bool)
            n239 = Select(t=Climber."ELEVATE!", s=w481, f=w484) -> (s? t:f=w485:T1)
          }
          frame "ELEVATE!" {
            n240 = global read "Robot Global Data.vi" "Climber Encoder"() -> (w500:dbl)
            n241 = global read "Robot Global Data.vi" "Climber Limit"() -> (w495:bool)
            n242 = Greater?(x=w500, y="Front Limit") -> (0:w496:bool)
            n243 = And(x=w496, y=w495) -> (x .and. y?=w494:bool)
            n244 = Select(t="Break speed", s=w496, f="Front Speed") -> (s? t:f=w502:dbl)
            n245 = Select(t="Break speed", s=w495, f="Back Speed") -> (s? t:f=w504:dbl)
            n246 = Select(t=Climber."Hold position", s=w494, f=w497) -> (s? t:f=w498:T1)
          }
          frame "Hold position" {
            n247 = global read "Robot Global Data.vi" "Buttons - Joy 0"() -> (w508:T10)
            n248 = Unbundle By Name(w508) -> ("Buttons[2]"=w507:bool)
            n249 = Select(t=Climber."Forward", s=w507, f=w509) -> (s? t:f=w510:T1)
            n250 = local read "Break speed"() -> (w511:dbl)
          }
          frame "Forward" {
            n251 = global read "Robot Global Data.vi" "Buttons - Joy 0"() -> (w514:T10)
            n252 = Unbundle By Name(w514) -> ("Buttons[3]"=w513:bool)
            n253 = Select(t=Climber."Retract varetas", s=w513, f=w517) -> (s? t:f=w518:T1)
            n254 = local read "Break speed"() -> (w519:dbl)
          }
          frame "Retract varetas" {
            n255 = global read "Robot Global Data.vi" "Climber Encoder"() -> (w528:dbl)
            n256 = Greater?(x=w528, y="Retract Distance") -> (0:w524:bool)
            n257 = Select(t=Climber."Charge", s=w524, f=w525) -> (s? t:f=w526:T1)
          }
          frame "Charge" {
            w541 = 0.4
            n258 = global read "Robot Global Data.vi" "Buttons - Joy 0"() -> (w537:T10)
            n259 = Unbundle By Name(w537) -> ("Buttons[1]"=w536:bool, "Buttons[2]"=w531:bool)
            n260 = Select(t=Climber."Sobe so um poquinho", s=w536, f=w539) -> (s? t:f=w540:T1)
            n261 = Select(t=0.9, s=w531, f=0.0) -> (s? t:f=w534:dbl)
          }
          frame "Sobe so um poquinho" {
            n262 = Increment(x=w547) -> (x+1=w546:dbl)
            n263 = Greater?(x=w546, y=10.0) -> (0:w548:bool)
            n264 = Select(t=Climber."cabou", s=w548, f=w549) -> (s? t:f=w550:T1)
          }
          frame "cabou" {
            # "É nois valeu falou"
          }
        }
        n265 = call <vilib>:"WPI_JoystickRefNum Registry Get.vi"("refnum name"="Joystick 0") -> ("error out"=w446:errorcluster, "JoystickDevRef"=w447:T27)  [unwired: 9 in]
        n266 = global write "Robot Global Data.vi" "Back Speed"(w453) -> ()
        n267 = global write "Robot Global Data.vi" "Front Speed"(w452) -> ()
        n268 = Wait (ms)(milliseconds to wait=u32 100) -> ()  [unwired: 1 out]
        n269 = global write "Robot Global Data.vi" "Climber Pivot"(w444) -> ()
        n270 = global write "Robot Global Data.vi" "Reset Climber Encoder"(w443) -> ()
        n271 = global write "Robot Global Data.vi" "Climber Enabled"(w439) -> ()
        n272 = call <vilib>:"WPI_JoystickSetOutputs.vi"("error in (no error)"=w446, "Right Rumble"=w448, "Left Rumble"=w449, "JoystickDevRef"=w447) -> ()  [unwired: 6 in, 2 out]
        "Climber State" <- w456
      }
    }
    frame Enabled {
      w554 = 0.0
      n273 = while {
        shift-right: [w573] -> _
        shift-left: Climber."Wait for Start" -> [w575]
        shift-right: [w569] -> _
        shift-left: w554 -> [w570]
        shift-right: [w556] -> _
        shift-left: w554 -> [w557]
        stop <- FALSE stop-if-true
        n274 = call <vilib>:"WPI_CompressorRefNum Registry Get.vi"("refnum name"="Compressor") -> ("error out"=w560:errorcluster, "CompressorDevRef"=w561:T26)  [unwired: 9 in]
        n275 = case shown="\"cabou\"" w575 {
          selector: w575 -> [w589 w603 w619 w631 w639 w647 w661 w671 _]
          tunnel: [w590 w604 w620 w632 w640 w648 w662 w672 Climber."cabou"] -> w573
          tunnel: [w586 _ w626 w633 w641 _ w656 "Retract back Speed 2" _] -> w572
          tunnel: [w586 _ w624 w633 w641 "Retract Speed 2" _ _ _] -> w571
          tunnel: w570 -> [_ w609 _ _ _ _ _ w669 _]
          tunnel: [_ w608 _ _ _ _ _ w668 _] -> w569
          tunnel: [w580 0.6 _ _ _ _ w663 _ _] -> w568
          tunnel: [w580 0.6 _ _ _ _ w663 _ _] -> w567
          tunnel: [_ _ _ _ TRUE TRUE TRUE TRUE TRUE] -> w563
          tunnel: [FALSE TRUE _ _ TRUE _ _ _ _] -> w562
          tunnel: w561 -> [_ w596 _ _ _ _ _ _ _]
          tunnel: w560 -> [_ w595 _ _ _ _ _ _ _]
          tunnel: [_ TRUE TRUE TRUE TRUE TRUE TRUE TRUE _] -> w558
          tunnel: w557 -> [_ _ w613 _ _ _ _ _ _]
          tunnel: [_ _ w612 _ _ _ _ _ _] -> w556
          frame "Wait for Start", Default {
            w586 = 0.0
            n276 = global read "Robot Global Data.vi" "Buttons - Joy 0"() -> (w593:T10)
            n277 = Unbundle By Name(w593) -> ("Buttons[6]"=w592:bool, "Buttons[7]"=w591:bool)
            n278 = global read "Robot Global Data.vi" "Robot Mode"() -> (w584:T25)
            n279 = global read "Robot Global Data.vi" "Rumble"() -> (w581:bool)
            n280 = And(x=w592, y=w591) -> (x .and. y?=w587:bool)
            n281 = Equal?(x=w584, y=WPI_DriverStationRobotMode2."Autonomous Enabled") -> (x = y?=w582:bool)
            n282 = And(x=w582, y=w581) -> (x .and. y?=w579:bool)
            n283 = Select(t=Climber."Engaging Climb", s=w587, f=w589) -> (s? t:f=w590:T1)
            n284 = Select(t=0.6, s=w579, f=0.0) -> (s? t:f=w580:dbl)
          }
          frame "Engaging Climb" {
            n285 = call <vilib>:"WPI_CompressorStop.vi"("error in (no error)"=w595, "CompressorDevRef"=w596) -> ()  [unwired: 8 in, 2 out]
            n286 = global read "Robot Global Data.vi" "Buttons - Joy 0"() -> (w601:T10)
            n287 = Unbundle By Name(w601) -> ("Buttons[0]"=w598:bool)
            n288 = Increment(x=w609) -> (x+1=w608:dbl)
            n289 = Greater?(x=w608, y=2.0) -> (0:w599:bool)
            n290 = And(x=w598, y=w599) -> (x .and. y?=w600:bool)
            n291 = Select(t=Climber."ELEVATE!", s=w600, f=w603) -> (s? t:f=w604:T1)
          }
          frame "ELEVATE!" {
            n292 = global read "Robot Global Data.vi" "Climber Encoder"() -> (w622:dbl)
            n293 = Increment(x=w613) -> (x+1=w612:dbl)
            n294 = Greater?(x=w622, y="Front Limit 2") -> (0:w618:bool)
            n295 = Greater?(x=w612, y="Back Timer") -> (0:w610:bool)
            n296 = And(x=w618, y=w610) -> (x .and. y?=w617:bool)
            n297 = Select(t="Break speed 2", s=w618, f="Front Speed 2") -> (s? t:f=w624:dbl)
            n298 = Select(t="Break speed 2", s=w610, f="Back Speed 2") -> (s? t:f=w626:dbl)
            n299 = Select(t=Climber."Hold position", s=w617, f=w619) -> (s? t:f=w620:T1)
          }
          frame "Hold position" {
            n300 = global read "Robot Global Data.vi" "Buttons - Joy 0"() -> (w630:T10)
            n301 = Unbundle By Name(w630) -> ("Buttons[2]"=w629:bool)
            n302 = Select(t=Climber."Forward", s=w629, f=w631) -> (s? t:f=w632:T1)
            n303 = local read "Break speed 2"() -> (w633:dbl)
          }
          frame "Forward" {
            n304 = global read "Robot Global Data.vi" "Buttons - Joy 0"() -> (w636:T10)
            n305 = Unbundle By Name(w636) -> ("Buttons[3]"=w635:bool)
            n306 = Select(t=Climber."Retract varetas", s=w635, f=w639) -> (s? t:f=w640:T1)
            n307 = local read "Break speed 2"() -> (w641:dbl)
          }
          frame "Retract varetas" {
            n308 = global read "Robot Global Data.vi" "Climber Encoder"() -> (w650:dbl)
            n309 = Greater?(x=w650, y="Retract Distance 2") -> (0:w646:bool)
            n310 = Select(t=Climber."Charge", s=w646, f=w647) -> (s? t:f=w648:T1)
          }
          frame "Charge" {
            w663 = 0.4
            n311 = global read "Robot Global Data.vi" "Buttons - Joy 0"() -> (w659:T10)
            n312 = Unbundle By Name(w659) -> ("Buttons[1]"=w658:bool, "Buttons[2]"=w653:bool)
            n313 = Select(t=Climber."Sobe so um poquinho", s=w658, f=w661) -> (s? t:f=w662:T1)
            n314 = Select(t=0.9, s=w653, f=0.0) -> (s? t:f=w656:dbl)
          }
          frame "Sobe so um poquinho" {
            n315 = Increment(x=w669) -> (x+1=w668:dbl)
            n316 = Greater?(x=w668, y=10.0) -> (0:w670:bool)
            n317 = Select(t=Climber."cabou", s=w670, f=w671) -> (s? t:f=w672:T1)
          }
          frame "cabou" {
            # "É nois valeu falou"
          }
        }
        n318 = call <vilib>:"WPI_JoystickRefNum Registry Get.vi"("refnum name"="Joystick 0") -> ("error out"=w565:errorcluster, "JoystickDevRef"=w566:T27)  [unwired: 9 in]
        n319 = global write "Robot Global Data.vi" "Back Speed"(w572) -> ()
        n320 = global write "Robot Global Data.vi" "Front Speed"(w571) -> ()
        n321 = Wait (ms)(milliseconds to wait=u32 100) -> ()  [unwired: 1 out]
        n322 = global write "Robot Global Data.vi" "Climber Pivot"(w563) -> ()
        n323 = global write "Robot Global Data.vi" "Reset Climber Encoder"(w562) -> ()
        n324 = global write "Robot Global Data.vi" "Climber Enabled"(w558) -> ()
        n325 = call <vilib>:"WPI_JoystickSetOutputs.vi"("error in (no error)"=w565, "Right Rumble"=w567, "Left Rumble"=w568, "JoystickDevRef"=w566) -> ()  [unwired: 6 in, 2 out]
        "Climber State 2" <- w575
      }
    }
  }
